vi "NodosPropiedad_Graficas.vi"() -> ()   [LabVIEW 2020]
panel:
  in  "?":bool
  out "Out of Range":bool
  in  "High Limit":dbl
  in  "Sample Rate (ms)":dbl
  out "Points Acquired":dbl
  in  "Points to Acquire":dbl
  out "Data and Time":string
  out "Temperature":cluster{dbl, "High Limit":dbl}(graph)
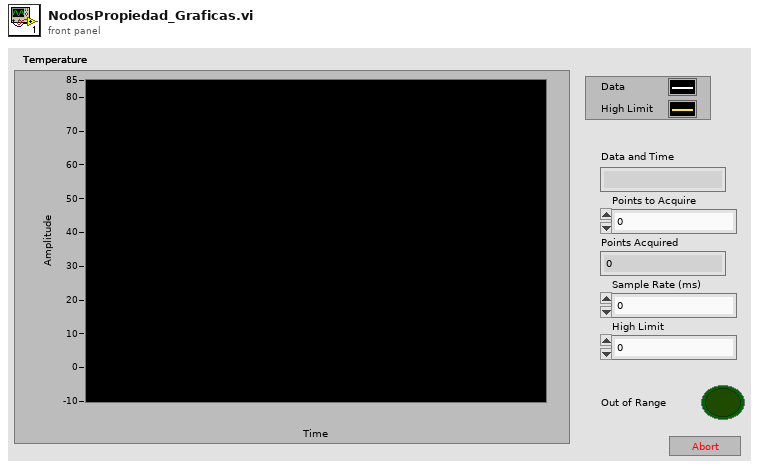
[diagram p1: front panel]
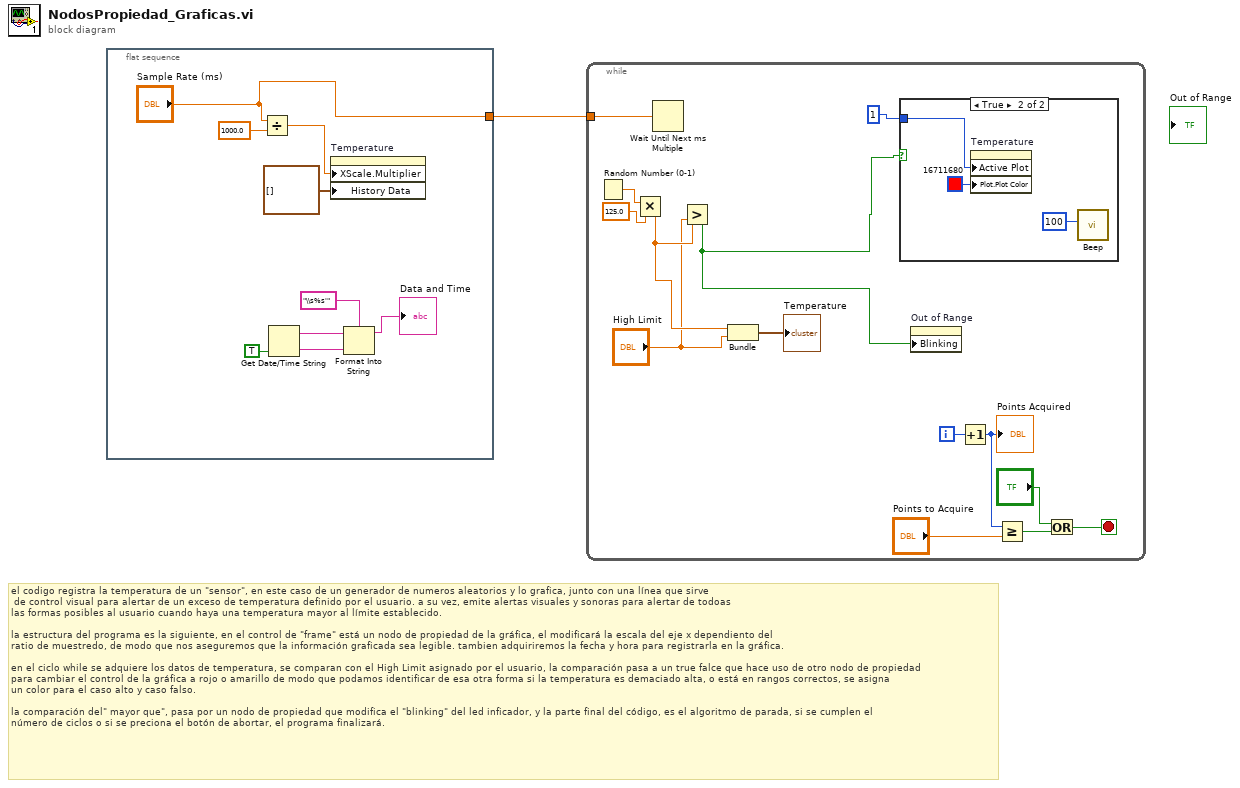
[diagram p0: block diagram]
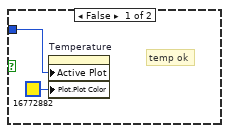
[diagram p2: hidden frame]
diagram:
  # "el codigo registra la temperatura de un \"sensor\", en este caso de un generador de numeros aleatorios y lo grafica, junto con una línea que sirve\n de control visual para alertar de un exceso de temperatura definido por el usuario. a su vez, emite alertas visuales y sonoras para alertar de todoas \nlas formas posibles al usuario cuando haya una temperatura mayor al límite establecido. \n\nla estructura del programa es la siguiente, en el control de \"frame\" está un nodo de propiedad de la gráfica, el modificará la escala del eje x dependiento del\nratio de muestredo, de modo que nos aseguremos que la información graficada sea legible. tambien adquiriremos la fecha y hora para registrarla en la gráfica. \n\nen el ciclo while se adquiere los datos de temperatura, se comparan con el High Limit asignado por el usuario, la comparación pasa a un true falce que hace uso de otro nodo de propiedad\npara cambiar el control de la gráfica a rojo o amarillo de modo que podamos identificar de esa otra forma si la temperatura es demaciado alta, o está en rangos correctos, se asigna \nun color para el caso alto y caso falso. \n\nla comparación del\" mayor que\", pasa por un nodo de propiedad que modifica el \"blinking\" del led inficador, y la parte final del código, es el algoritmo de parada, si se cumplen el \nnúmero de ciclos o si se preciona el botón de abortar, el programa finalizará."
  n1 = flat-sequence {
    tunnel: ["Sample Rate (ms)"] -> w1
    frame #0 {
      n2 = Divide(x="Sample Rate (ms)", y=1000.0) -> (x/y=w4:dbl)
      n3 = Get Date/Time String(want seconds? (F)=TRUE) -> (date string=w9:string, time string=w8:string)  [unwired: 2 in]
      n4 = property on="Temperature" class="WFChart (strict)"("XScale.Multiplier"=w4, "History Data"=cluster{dbl, "High Limit":dbl}[] []) -> ()  [unwired: 2 in, 2 out]
      n5 = Format Into String "Format Into String"(format string="\\s%s'", initial string=w9, w8) -> (resulting string=→"Data and Time":string)  [unwired: 1 in, 1 out]
    }
  }
  n6 = while {
    tunnel: w1 -> [w24]
    i -> [w16]
    stop <- w11 stop-if-true
    n7 = Random Number (0-1)() -> (number: 0 to 1=w22:dbl)
    n8 = Multiply(x=w22, y=125.0) -> (x*y=w20:dbl)
    n9 = Wait Until Next ms Multiple(millisecond multiple=w24) -> ()  [unwired: 1 out]
    n10 = Greater?(x=w20, y="High Limit") -> (0:w18:bool)
    n11 = Bundle(w20, "High Limit"="High Limit") -> (→"Temperature":cluster{dbl, "High Limit":dbl})  [unwired: 1 in]
    n12 = case shown="True" w18 {
      tunnel: 1 -> [w25 w29]
      frame False {
        # "temp ok"
        n13 = property on="Temperature" class="WFChart (strict)"("Active Plot"=w25, "Plot.Plot Color"=u32 16772882) -> ()  [unwired: 2 in, 2 out]
      }
      frame True {
        n14 = property on="Temperature" class="WFChart (strict)"("Active Plot"=w29, "Plot.Plot Color"=u32 16711680) -> ()  [unwired: 2 in, 2 out]
        n15 = call <vilib>:"Beep.vi"("duration (msec)"=u32 100) -> ()  [unwired: 11 in]
      }
    }
    n16 = property on="Out of Range" class="Bool (strict)"("Blinking"=w18) -> ()  [unwired: 2 in, 2 out]
    n17 = Increment(x=w16) -> (x+1=w14:i32)
    "Points Acquired" <- w14
    n18 = Greater Or Equal?(x=w14, y="Points to Acquire") -> (x >= y?=w12:bool)
    n19 = Or(x="?", y=w12) -> (x .or. y?=w11:bool)
  }
